vi "digital output.vi"() -> ()   [LabVIEW 2011]
uses:
  <vilib>/platform/TimedLoop/XDataNode/XDataNode.xnode
  <vilib>/Platform/TimedLoop/XDataNode/nitl_modes.ctl
  <vilib>/Platform/TimedLoop/XDataNode/XDNodeRunTimeDep.lvlib
  <vilib>/Platform/TimedLoop/XDataNode/wakeup.ctl
  <vilib>/Platform/TimedLoop/XDataNode/timing_clust.ctl
  <vilib>/DAQmx/write.llb/DAQmx Write (Digital Bool 1Line 1Point).vi
  <vilib>/Platform/TimedLoop/scheduler/LVUserAPI/_suppVIs/Create_1kHz_TSource.vi
panel:
  in  "train length (ms)":i64=2000
  in  "send":bool
  in  "stop":bool
  out "Digital Waveform Graph":digitalwaveform(graph)
  in  "percent for random":dbl=20.0
  in  "nominal freq (Hz)":i32=20
  in  "DO duration (ms)":i32=1000
  in  "H duration (ms)":i32=10
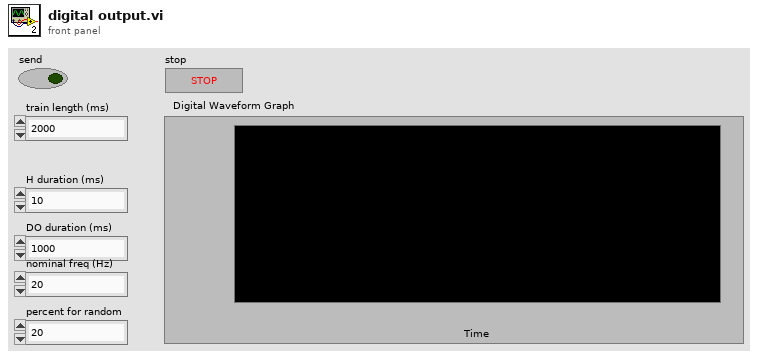
[diagram p1: front panel]
types:
  T1 = typedef "XDNodeRunTimeDep.lvlib/timing_clust.ctl" = cluster{"Expected End [f-1]":u64, "Actual End [f-1]":u64, "Finished Late? [f-1]":bool, "Expected End [i-1]":u64, "Actual End [i-1]":u64, "Finished Late? [i-1]":bool, "Expected Start [i]":u64, "Actual Start [i]":u64, "Expected Start [f]":u64, "Actual Start [f]":u64, "Source Name":string, "Structure Name":string, "Period":i64, "Deadline":i64, "Offset":i64, "Start":i64, "Priority":i32, "Timeout":i32, "Mode":T2, "Wakeup Reason":T3, "Error":errorcluster, "Source Type":string, "Secondary Source Type":string, "Global End Time":u64, "Global Start Time":u64, "Frame Duration":u64, "Iteration Duration":u64, "Assigned CPU":i32, "I/O Scan Engine Mode":u32}
  T2 = typedef "XDNodeRunTimeDep.lvlib/nitl_modes.ctl" = enum32{"No Change", "Process missed periods, maintain original phase", "Discard missed periods, maintain original phase", "Process missed periods, ignore original phase", "Discard missed periods, ignore original phase"}
  T3 = typedef "XDNodeRunTimeDep.lvlib/wakeup.ctl" = enum32{"Normal", "Aborted", "Asynchronous wakeup", "Timing source error", "Timed loop error", "Timeout"}
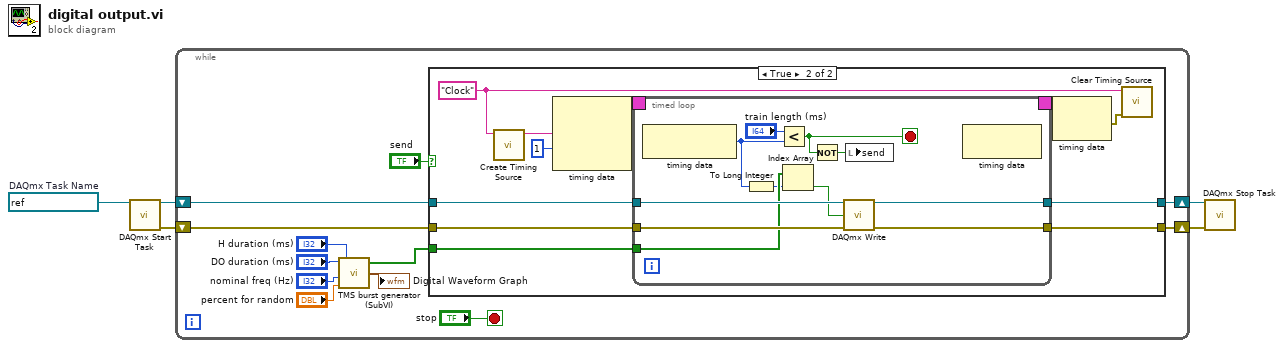
[diagram p0: block diagram]
diagram:
  w5 = refnum<k21> "RandomDO"  # DAQmx Task Name
  n1 = call <vilib>:"DAQmx Start Task.vi"("task/channels in"=w5) -> ("task out"=w4:refnum<k21>, "error out"=w2:errorcluster)  [unwired: 13 in]
  n2 = while {
    shift-right: [w16] -> w3
    shift-left: w4 -> [w17]
    shift-right: [w14] -> w1
    shift-left: w2 -> [w15]
    stop <- "stop" stop-if-true
    n3 = call "TMS burst generator (SubVI).vi"("percent for random"="percent for random", "nominal freq (Hz)"="nominal freq (Hz)", "H duration (ms)"="H duration (ms)", "Total duration (ms)"="DO duration (ms)") -> ("digital waveform"=→"Digital Waveform Graph":digitalwaveform, "out"=w6:bool[])  [unwired: 1 out]
    n4 = case shown="True" "send" {
      tunnel: w17 -> [w19 w28]
      tunnel: [w19 w27] -> w16
      tunnel: w15 -> [w18 w26]
      tunnel: [w18 w25] -> w14
      tunnel: w6 -> [_ w23]
      frame False {
      }
      frame True {
        w20 = "Clock" ("name (in)")
        n5 = call-poly <vilib>:"Create Timing Source.vi"("name (in)"=w20) -> ("name (out)"=w22:string)  [unwired: 9 in, 1 out]
        n6 = node-c288(w22, i64 1 ("Period")) -> (w30:T1)  [unwired: 1 in]
        n7 = timed-loop {
          tunnel: w28 -> [w41]
          tunnel: [w40] -> w27
          tunnel: w26 -> [w39]
          tunnel: [w38] -> w25
          timing: w30 -> [_]
          timing-out: [_] -> w29
          tunnel: w23 -> [w37]
          stop <- w34 stop-if-true
          n8 = node-c288() -> (w32:i64)  [unwired: 1 in]
          n9 = To Long Integer(number=w32) -> (32bit integer=w35:i32)
          n10 = Less?(x="train length (ms)", y=w32) -> (x < y?=w34:bool)
          n11 = Index Array(array=w37, index=w35) -> (element=w36:bool)
          n12 = Not(x=w34) -> (.not. x?=w33:bool)
          n13 = call-poly <vilib>:"DAQmx Write.vi"("task/channels in"=w41, "data"=w36, "error in"=w39) -> ("task out"=w40:refnum<k21>, "error out"=w38:errorcluster)  [unwired: 10 in, 1 out]
          n14 = local write "send"(w33) -> ()
          n15 = node-c288() -> ()  [unwired: 1 in, 1 out]
        }
        n16 = node-c288(w29) -> (w21:errorcluster)
        n17 = call <vilib>:"Clear Timing Source.vi"("error in (no error)"=w21, "name"=w20) -> ()  [unwired: 8 in, 2 out]
      }
    }
  }
  n18 = call <vilib>:"DAQmx Stop Task.vi"("task/channels in"=w3, "error in"=w1) -> ()  [unwired: 12 in, 2 out]
